vi "libssh2_sftp_mkdir_ex.vi"(7 "mode":i32(ring) items=["LIBSSH2_SFTP_S_IRWXU"=448, "LIBSSH2_SFTP_S_IRUSR"=256, "LIBSSH2_SFTP_S_IWUSR"=128, "LIBSSH2_SFTP_S_IXUSR"=64, "LIBSSH2_SFTP_S_IRWXG"=56, "LIBSSH2_SFTP_S_IRGRP"=32, "LIBSSH2_SFTP_S_IWGRP"=16, "LIBSSH2_SFTP_S_IXGRP"=8, "LIBSSH2_SFTP_S_IRWXO"=7, "LIBSSH2_SFTP_S_IROTH"=4, "LIBSSH2_SFTP_S_IWOTH"=2, "LIBSSH2_SFTP_S_IXOTH"=1], 8 "error in (no error)":errorcluster, 10 "path":string, 11 "sftp":T1) -> (0 "error out":errorcluster)   [LabVIEW 2017, in "libssh2.lvlib"]
doc: "Create a directory with custom permissions."
uses:
  libssh2.lvlib
  SFTP Refnum.ctl
  Acquire Session.vi
  Release Session.vi
  Not An SFTP Refnum.vi
  <vilib>/Utility/error.llb/Error Cluster From Error Code.vi
  Global Settings.vi
  Read SFTP Refnum.vi
  Read Session Refnum.vi
  <vilib>/Utility/semaphor.llb/Acquire Semaphore.vi
  <vilib>/Utility/semaphor.llb/Release Semaphore.vi
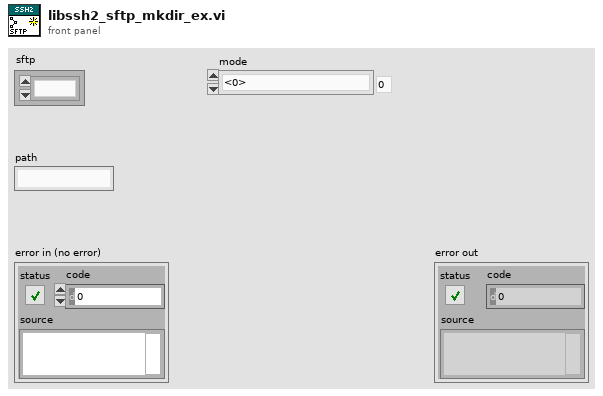
[diagram p1: front panel]
types:
  T1 = typedef "libssh2.lvlib/SFTP Refnum.ctl" = refnum<k1>
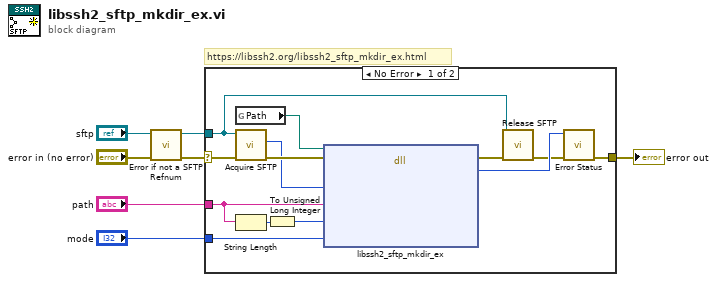
[diagram p0: block diagram]
diagram:
  # "https://libssh2.org/libssh2_sftp_mkdir_ex.html"
  n1 = call "Error if not a SFTP Refnum.vi"("error in (no error)"="error in (no error)", "sftp"="sftp") -> ("error out"=w6:errorcluster, "sftp out"=w5:T1)  [unwired: 8 in]
  n2 = case shown="No Error" w6 {
    selector: w6 -> [w19 w21]
    tunnel: w5 -> [w8 _]
    tunnel: [w15 w21] -> w4
    tunnel: "path" -> [w13 _]
    tunnel: "mode" -> [w10 _]
    frame No Error {
      n3 = global read "Global Settings.vi" "Path"() -> (w20:path)
      n4 = call "Acquire SFTP.vi"("error in (no error)"=w19, "sftp"=w8) -> ("error out"=w18:errorcluster, "LIBSSH2_SFTP*"=w17:u64)  [unwired: 8 in]
      n5 = String Length(string=w13) -> (length=w12:i32)
      n6 = To Unsigned Long Integer(number=w12) -> (unsigned 32bit integer=w11:u32)
      n7 = dll-call lib="?" fn="libssh2_sftp_mkdir_ex"(path in=w20, error in=w18, "sftp"=w17, "path"=w13, "path_len"=w11, "mode"=w10) -> (error out=w16:errorcluster, "return value"=w14:i32)  [unwired: 5 in, 1 out]
      n8 = call "Release SFTP.vi"("error in (no error)"=w16, "sftp"=w8) -> ("error out"=w9:errorcluster)  [unwired: 9 in]
      n9 = call "Error Status.vi"("error in (no error)"=w9, "return value"=w14) -> ("error out"=w15:errorcluster)  [unwired: 8 in, 1 out]
    }
    frame Error {
    }
  }
  "error out" <- w4
